vi "AlarmasHMI.vi"() -> ()   [LabVIEW 2018]
uses:
  <vilib>/RAFA Solutions/Harmony UI Controls Kit/String & Path/String Indicator.ctl
  <vilib>/RAFA Solutions/Harmony UI Controls Kit/Boolean/OK Button.ctl
  <vilib>/RAFA Solutions/Harmony UI Controls Kit/List, Table & Tree/Multicolumn Listbox.ctl
  <vilib>/RAFA Solutions/Harmony UI Controls Kit/Boolean/Blank Button - Green.ctl
  Controls/Cluster_Alarmas_IEEE45.ctl
  <vilib>/RAFA Solutions/Harmony UI Controls Kit/Boolean/Round Led.ctl
  Controls/Hora y Fecha control.ctl
  Global/globalEventos.vi
  Global/Alarmas_indicadores-LED.vi
  <vilib>/addons/database/Connection.llb/DB Tools Open Connec (Path).vi
  Global/AlarmasGlobal.vi
  <vilib>/RAFA Solutions/Harmony UI Controls Kit/Flat UI Design.lvlib
  <vilib>/addons/database/NI_Database_API.lvlib
panel:
  out "fecha y hora":T1
  out "G6_TRANS":T2 caption="Transiente"
  out "G6_SWELL":T2 caption="Swell"
  out "G6_SAG":T2 caption="Sag"
  out "G5_TRANS":T2 caption="Transiente"
  out "G5_SWELL":T2 caption="Swell"
  out "G5_SAG":T2 caption="Sag"
  out "G4_TRANS":T2 caption="Transiente"
  out "G4_SWELL":T2 caption="Swell"
  out "G4_SAG":T2 caption="Sag"
  out "G3_TRANS":T2 caption="Transiente"
  out "G3_SWELL":T2 caption="Swell"
  out "G3_SAG":T2 caption="Sag"
  out "G2_TRANS":T2 caption="Transiente"
  out "G2_SWELL":T2 caption="Swell"
  out "G2_SAG":T2 caption="Sag"
  out "G1_TRANS":T2 caption="Transiente"
  out "G1_SWELL":T2 caption="Swell"
  out "G1_SAG":T2 caption="Sag"
  out "Generador 6":T3={"V1_V2 (V) "={0.0, 17.0, 16.662651515468255}, "Mod_V1_V2"=0.0, "alarma 1"=FALSE, "Mod_V2_V3"=0.0, "alarma 2"=FALSE, "Mod_V3_V1"=0.0, "alarma 3"=FALSE, "Mod_Frec"=0.0, "alarma 4"=FALSE, "V2_V3 (V)"={0.0, 17.0, 16.662651515468255}, "V3_V1 (V)"={0.0, 17.0, 16.662651515468255}, "Frecuencia (Hz)"={0.0, 17.0, 16.662651515468255}, "AVG VL_VL (V)"={0.0, 17.0, 16.662651515468255}, "alarm 5"=FALSE, "alarm 6"=FALSE, "alarm 7"=FALSE, "alarm 8"=FALSE, "alarm 9"=FALSE} {"AVG VL_VL (V)" scale=427.0..473.0; "Frecuencia (Hz)" scale=58.0..62.0; "V3_V1 (V)" scale=418.0..482.0; "V2_V3 (V)" scale=418.0..482.0; "Mod_Frec" format="%#.1f"; "Mod_V3_V1" format="%#.1f"; "Mod_V2_V3" format="%#.1f"; "Mod_V1_V2" format="%#.1f"; "V1_V2 (V)" scale=418.0..482.0}
  out "Generador 5":T3={"V1_V2 (V) "={0.0, 17.0, 16.662651515468255}, "Mod_V1_V2"=0.0, "alarma 1"=FALSE, "Mod_V2_V3"=0.0, "alarma 2"=FALSE, "Mod_V3_V1"=0.0, "alarma 3"=FALSE, "Mod_Frec"=0.0, "alarma 4"=FALSE, "V2_V3 (V)"={0.0, 17.0, 16.662651515468255}, "V3_V1 (V)"={0.0, 17.0, 16.662651515468255}, "Frecuencia (Hz)"={0.0, 17.0, 16.662651515468255}, "AVG VL_VL (V)"={0.0, 17.0, 16.662651515468255}, "alarm 5"=FALSE, "alarm 6"=FALSE, "alarm 7"=FALSE, "alarm 8"=FALSE, "alarm 9"=FALSE} {"AVG VL_VL (V)" scale=427.0..473.0; "Frecuencia (Hz)" scale=58.0..62.0; "V3_V1 (V)" scale=418.0..482.0; "V2_V3 (V)" scale=418.0..482.0; "Mod_Frec" format="%#.1f"; "Mod_V3_V1" format="%#.1f"; "Mod_V2_V3" format="%#.1f"; "Mod_V1_V2" format="%#.1f"; "V1_V2 (V)" scale=418.0..482.0}
  out "Generador 4":T3={"V1_V2 (V) "={0.0, 17.0, 16.662651515468255}, "Mod_V1_V2"=0.0, "alarma 1"=FALSE, "Mod_V2_V3"=0.0, "alarma 2"=FALSE, "Mod_V3_V1"=0.0, "alarma 3"=FALSE, "Mod_Frec"=0.0, "alarma 4"=FALSE, "V2_V3 (V)"={0.0, 17.0, 16.662651515468255}, "V3_V1 (V)"={0.0, 17.0, 16.662651515468255}, "Frecuencia (Hz)"={0.0, 17.0, 16.662651515468255}, "AVG VL_VL (V)"={0.0, 17.0, 16.662651515468255}, "alarm 5"=FALSE, "alarm 6"=FALSE, "alarm 7"=FALSE, "alarm 8"=FALSE, "alarm 9"=FALSE} {"AVG VL_VL (V)" scale=427.0..473.0; "Frecuencia (Hz)" scale=58.0..62.0; "V3_V1 (V)" scale=418.0..482.0; "V2_V3 (V)" scale=418.0..482.0; "Mod_Frec" format="%#.1f"; "Mod_V3_V1" format="%#.1f"; "Mod_V2_V3" format="%#.1f"; "Mod_V1_V2" format="%#.1f"; "V1_V2 (V)" scale=418.0..482.0}
  out "Generador 3":T3={"V1_V2 (V) "={0.0, 17.0, 16.662651515468255}, "Mod_V1_V2"=0.0, "alarma 1"=FALSE, "Mod_V2_V3"=0.0, "alarma 2"=FALSE, "Mod_V3_V1"=0.0, "alarma 3"=FALSE, "Mod_Frec"=0.0, "alarma 4"=FALSE, "V2_V3 (V)"={0.0, 17.0, 16.662651515468255}, "V3_V1 (V)"={0.0, 17.0, 16.662651515468255}, "Frecuencia (Hz)"={0.0, 17.0, 16.662651515468255}, "AVG VL_VL (V)"={0.0, 17.0, 16.662651515468255}, "alarm 5"=FALSE, "alarm 6"=FALSE, "alarm 7"=FALSE, "alarm 8"=FALSE, "alarm 9"=FALSE} {"AVG VL_VL (V)" scale=427.0..473.0; "Frecuencia (Hz)" scale=58.0..62.0; "V3_V1 (V)" scale=418.0..482.0; "V2_V3 (V)" scale=418.0..482.0; "Mod_Frec" format="%#.1f"; "Mod_V3_V1" format="%#.1f"; "Mod_V2_V3" format="%#.1f"; "Mod_V1_V2" format="%#.1f"; "V1_V2 (V)" scale=418.0..482.0}
  out "Generador 2":T3={"V1_V2 (V) "={0.0, 17.0, 16.662651515468255}, "Mod_V1_V2"=0.0, "alarma 1"=FALSE, "Mod_V2_V3"=0.0, "alarma 2"=FALSE, "Mod_V3_V1"=0.0, "alarma 3"=FALSE, "Mod_Frec"=0.0, "alarma 4"=FALSE, "V2_V3 (V)"={0.0, 17.0, 16.662651515468255}, "V3_V1 (V)"={0.0, 17.0, 16.662651515468255}, "Frecuencia (Hz)"={0.0, 17.0, 16.662651515468255}, "AVG VL_VL (V)"={0.0, 17.0, 16.662651515468255}, "alarm 5"=FALSE, "alarm 6"=FALSE, "alarm 7"=FALSE, "alarm 8"=FALSE, "alarm 9"=FALSE} {"AVG VL_VL (V)" scale=427.0..473.0; "Frecuencia (Hz)" scale=58.0..62.0; "V3_V1 (V)" scale=418.0..482.0; "V2_V3 (V)" scale=418.0..482.0; "Mod_Frec" format="%#.1f"; "Mod_V3_V1" format="%#.1f"; "Mod_V2_V3" format="%#.1f"; "Mod_V1_V2" format="%#.1f"; "V1_V2 (V)" scale=418.0..482.0}
  out "Generador 1":T3={"V1_V2 (V) "={0.0, 17.0, 16.662651515468255}, "Mod_V1_V2"=0.0, "alarma 1"=FALSE, "Mod_V2_V3"=0.0, "alarma 2"=FALSE, "Mod_V3_V1"=0.0, "alarma 3"=FALSE, "Mod_Frec"=0.0, "alarma 4"=FALSE, "V2_V3 (V)"={0.0, 17.0, 16.662651515468255}, "V3_V1 (V)"={0.0, 17.0, 16.662651515468255}, "Frecuencia (Hz)"={0.0, 17.0, 16.662651515468255}, "AVG VL_VL (V)"={0.0, 17.0, 16.662651515468255}, "alarm 5"=FALSE, "alarm 6"=FALSE, "alarm 7"=FALSE, "alarm 8"=FALSE, "alarm 9"=FALSE} {"AVG VL_VL (V)" scale=427.0..473.0; "Frecuencia (Hz)" scale=58.0..62.0; "V3_V1 (V)" scale=418.0..482.0; "V2_V3 (V)" scale=418.0..482.0; "Mod_Frec" format="%#.1f"; "Mod_V3_V1" format="%#.1f"; "Mod_V2_V3" format="%#.1f"; "Mod_V1_V2" format="%#.1f"; "V1_V2 (V)" scale=418.0..482.0}
  in  "Tiempo Final Eventos":timestamp caption="Tiempo Final" format="%<%X\n%x>T"
  in  "Tiempo Inicio Eventos":timestamp caption="Tiempo Inicio" format="%<%X\n%x>T"
  in  "Consultar Alarma":T4
  out "Tabla de Alarmas":T5
  out "Generador":string
  in  "volver":T6
  out "Eventos":T7
  # "Sistema de Monitoreo de Calidad de Energía"
  # "Límites y valores según IEEE45"
  # "Límites y valores según IEEE45"
  # "EMCE G01"
  # "EMCE G03"
  # "EMCE G02"
  # "EMCE G04"
  # "EMCE W01"
  # "EMCE W02"
  # "ALARMAS CALIDAD DE ENERGIA\nEN50160"
  # "EMCE G03"
  # "EMCE G01"
  # "EMCE G02"
  # "EMCE W01"
  # "EMCE G04"
  # "EMCE W02"
  # "Tolerancias"
  # "Modulación"
  # "%"
  # "%"
  # "%"
  # "5 % máx."
  # "%"
  # "0,5 % máx."
  # "Tolerancias"
  # "Modulación"
  # "%"
  # "%"
  # "%"
  # "5 % máx."
  # "%"
  # "0,5 % máx."
  # "Tolerancias"
  # "Modulación"
  # "%"
  # "%"
  # "%"
  # "5 % máx."
  # "%"
  # "0,5 % máx."
  # "Tolerancias"
  # "Modulación"
  # "%"
  # "%"
  # "%"
  # "5 % máx."
  # "%"
  # "0,5 % máx."
  # "Tolerancias"
  # "Modulación"
  # "%"
  # "%"
  # "%"
  # "5 % máx."
  # "%"
  # "0,5 % máx."
  # "Tolerancias"
  # "Modulación"
  # "%"
  # "%"
  # "%"
  # "5 % máx."
  # "%"
  # "0,5 % máx."
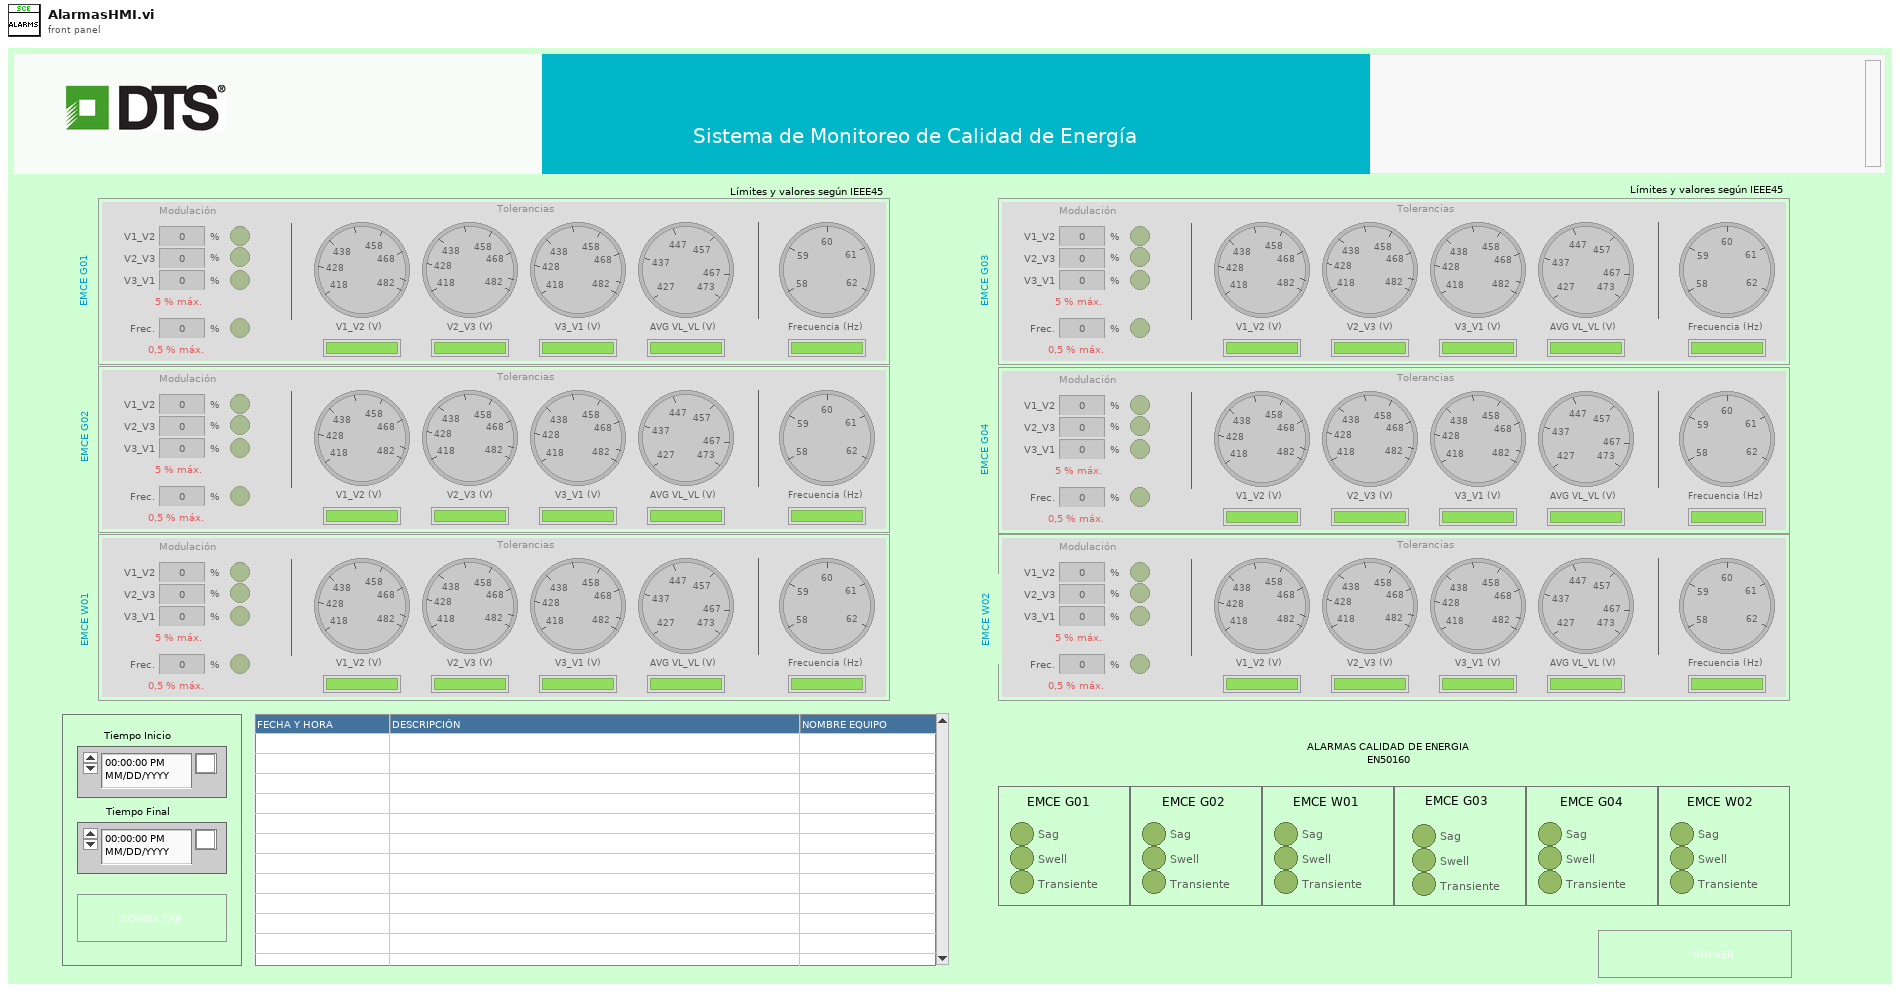
[diagram p1: front panel]
types:
  T1 = typedef "Hora y Fecha control.ctl" = cluster{"fecha":string, "dia semana":string, "fecha 2":string}
  T2 = typedef "Flat UI Design.lvlib/Round Led.ctl" = bool
  T3 = typedef "Cluster_Alarmas_IEEE45.ctl" = cluster{"V1_V2 (V) ":cluster{dbl, dbl, dbl}, "Mod_V1_V2":dbl, "alarma 1":T2, "Mod_V2_V3":dbl, "alarma 2":T2, "Mod_V3_V1":dbl, "alarma 3":T2, "Mod_Frec":dbl, "alarma 4":T2, "V2_V3 (V)":cluster{dbl, dbl, dbl}, "V3_V1 (V)":cluster{dbl, dbl, dbl}, "Frecuencia (Hz)":cluster{dbl, dbl, dbl}, "AVG VL_VL (V)":cluster{dbl, dbl, dbl}, "alarm 5":bool, "alarm 6":bool, "alarm 7":bool, "alarm 8":bool, "alarm 9":bool}
  T4 = typedef "Flat UI Design.lvlib/Blank Button - Green.ctl" = bool
  T5 = typedef "Flat UI Design.lvlib/Multicolumn Listbox.ctl" = i32
  T6 = typedef "Flat UI Design.lvlib/OK Button.ctl" = bool
  T7 = typedef "Flat UI Design.lvlib/String Indicator.ctl" = string
  T8 = typedef "NI_Database_API.lvlib/Conn ObjectReference.ctl" = refnum<k1>
  T9 = enum8{"Enabled", "Disabled", "Disabled and Grayed Out"}
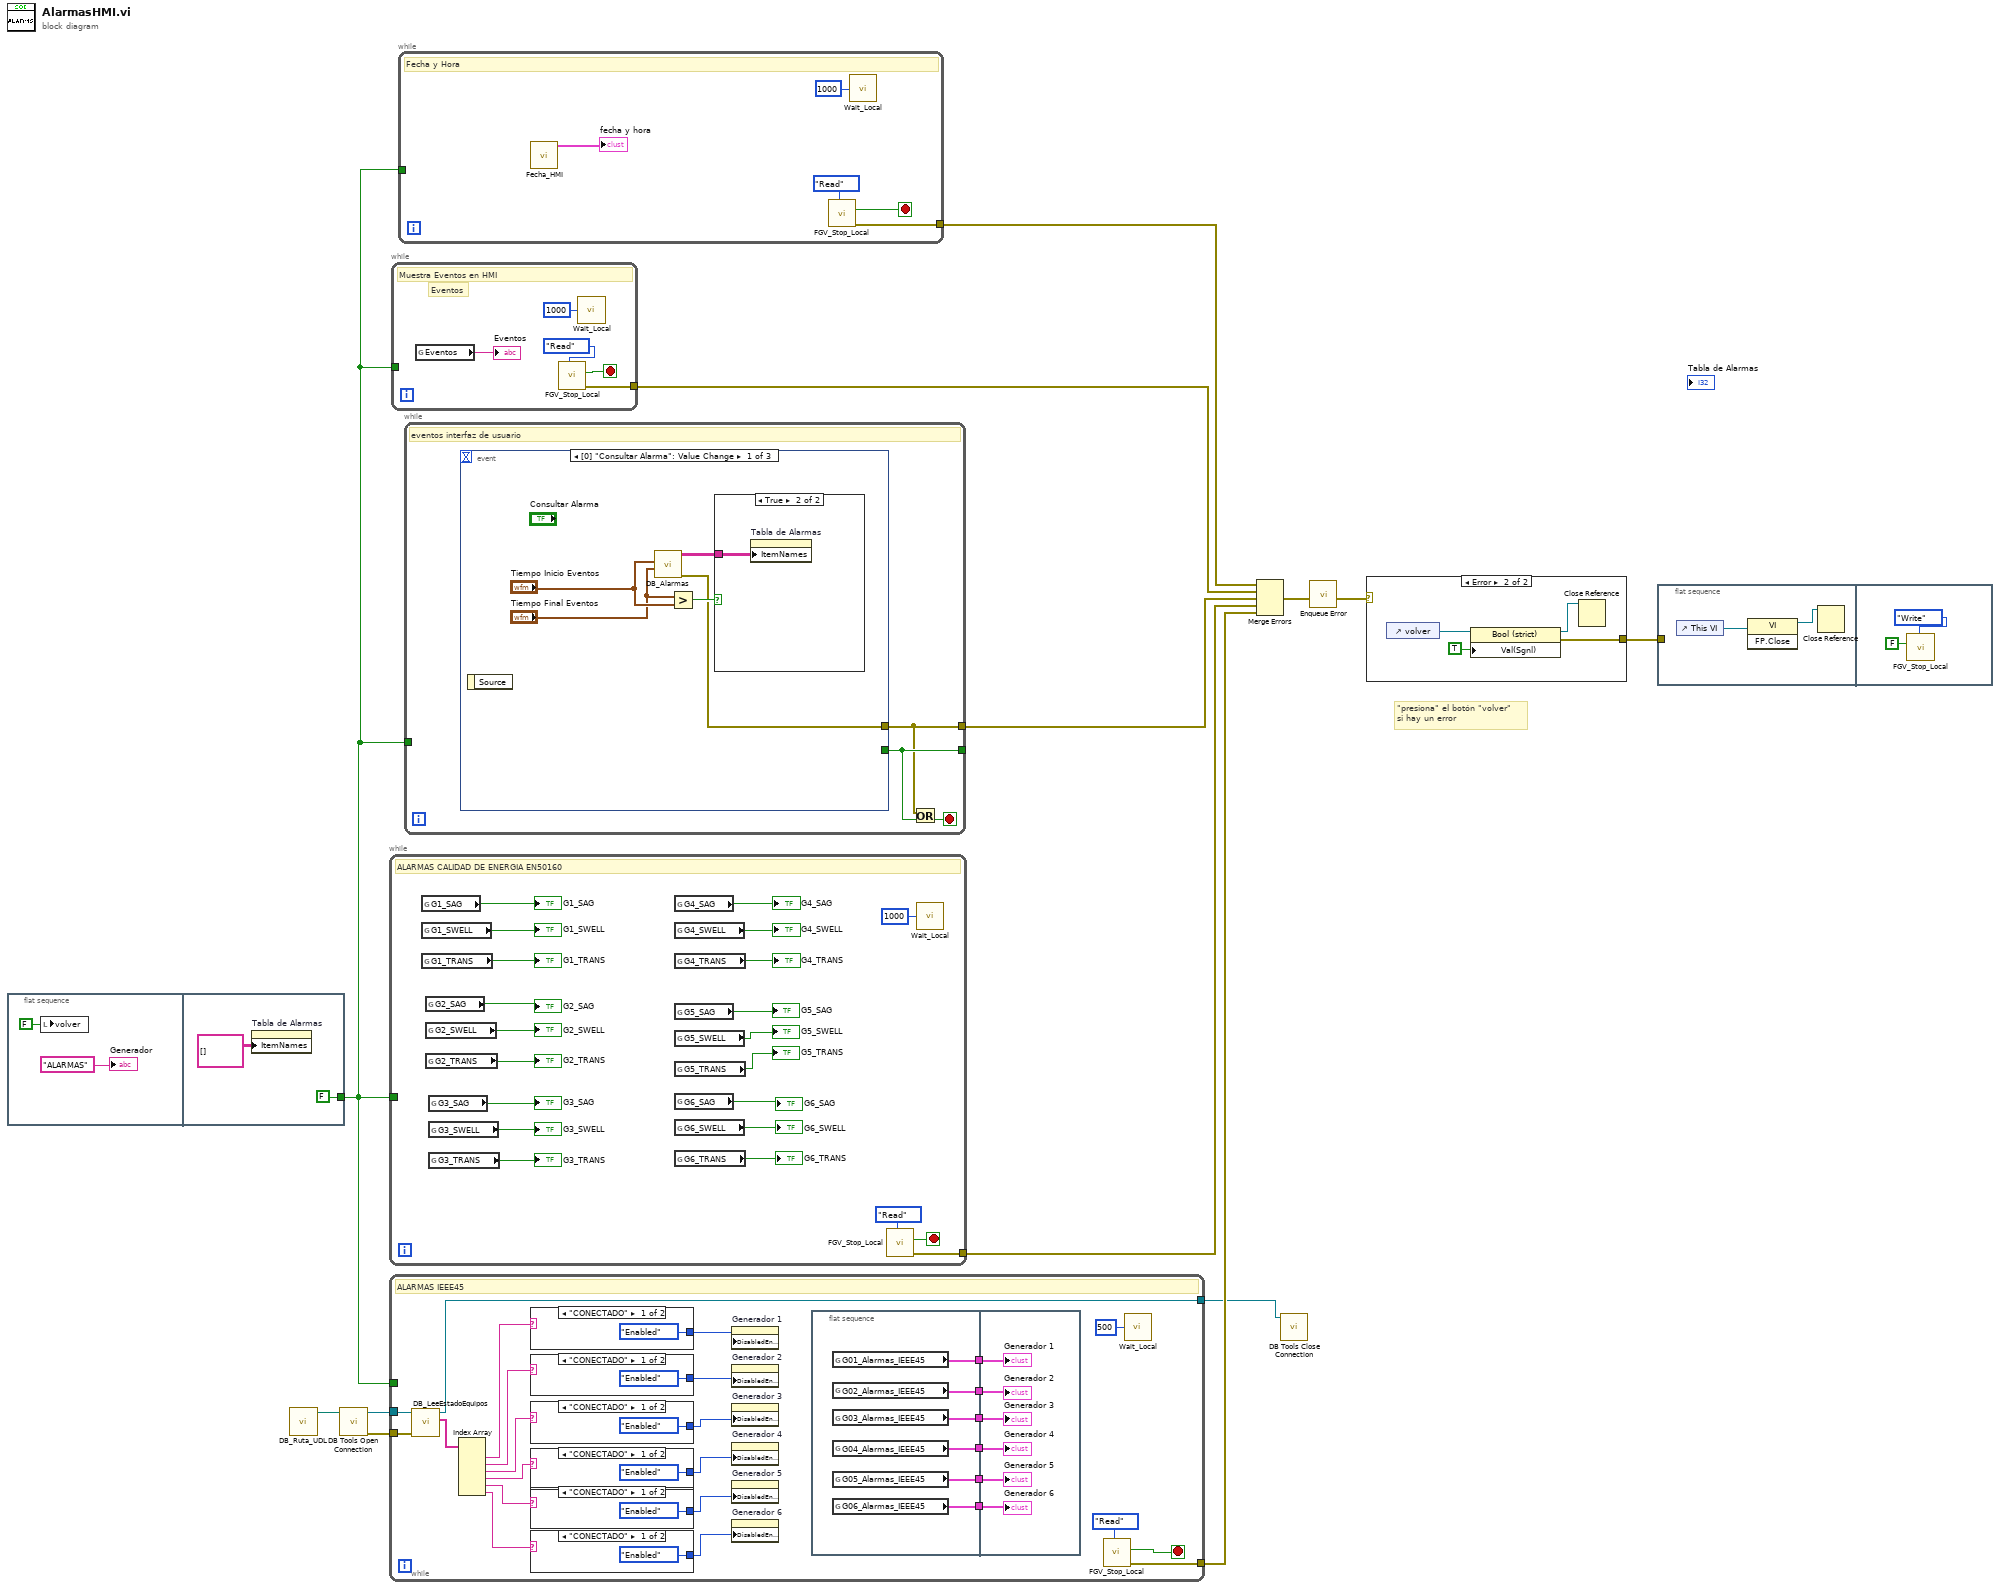
[diagram p0: block diagram]
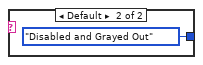
[diagram p3: hidden frame]
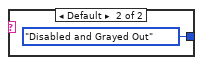
[diagram p4: hidden frame]
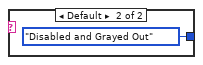
[diagram p5: hidden frame]
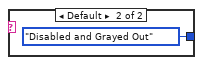
[diagram p6: hidden frame]
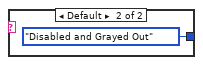
[diagram p7: hidden frame]
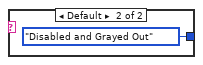
[diagram p8: hidden frame]
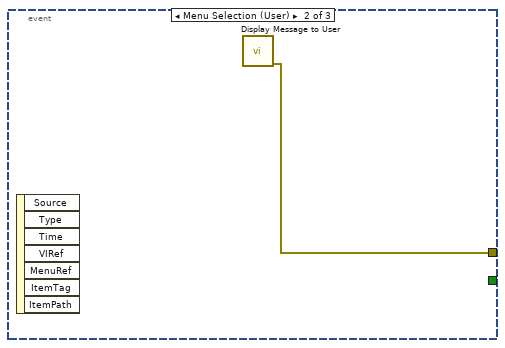
[diagram p10: hidden frame]
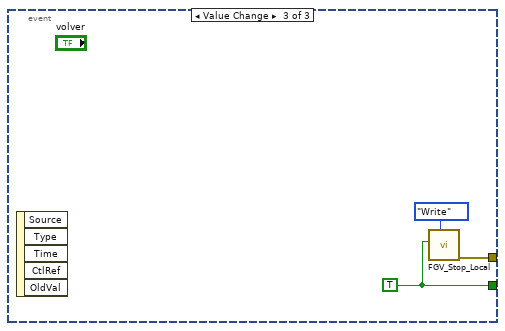
[diagram p11: hidden frame]
diagram:
  # "\"presiona\" el botón \"volver\"\nsi hay un error"
  n1 = flat-sequence {
    tunnel: [FALSE ("sag_flag")] -> w13
    frame #0 {
      n2 = local write "volver"(T6 FALSE ("volver")) -> ()
      "Generador" <- "ALARMAS" ("Generador in")
    }
    frame #1 {
      n3 = property on="Tabla de Alarmas" class="MCListbox (strict)"("ItemNames"=string[][] [] ("Item Names")) -> ()  [unwired: 2 in, 2 out]
    }
  }
  n4 = call "DB_Ruta_UDL.vi"() -> ("UDL ruta"=w4:path)  [unwired: 11 in]
  n5 = call-poly <vilib>:"DB Tools Open Connection.vi"("connection information"=w4) -> ("error out"=w3:errorcluster, "connection reference"=w2:T8)  [unwired: 7 in]
  n6 = while {
    tunnel: w13 -> [_]
    tunnel: [w36] -> w9
    stop <- w38 stop-if-true
    # "ALARMAS CALIDAD DE ENERGIA EN50160"
    n7 = global read "Alarmas_indicadores-LED.vi" "G1_SAG"() -> (→"G1_SAG":bool)
    n8 = global read "Alarmas_indicadores-LED.vi" "G1_SWELL"() -> (→"G1_SWELL":bool)
    n9 = global read "Alarmas_indicadores-LED.vi" "G1_TRANS"() -> (→"G1_TRANS":bool)
    n10 = global read "Alarmas_indicadores-LED.vi" "G2_SAG"() -> (→"G2_SAG":bool)
    n11 = global read "Alarmas_indicadores-LED.vi" "G2_SWELL"() -> (→"G2_SWELL":bool)
    n12 = global read "Alarmas_indicadores-LED.vi" "G2_TRANS"() -> (→"G2_TRANS":bool)
    n13 = global read "Alarmas_indicadores-LED.vi" "G3_SAG"() -> (→"G3_SAG":bool)
    n14 = global read "Alarmas_indicadores-LED.vi" "G3_SWELL"() -> (→"G3_SWELL":bool)
    n15 = global read "Alarmas_indicadores-LED.vi" "G3_TRANS"() -> (→"G3_TRANS":bool)
    n16 = global read "Alarmas_indicadores-LED.vi" "G4_SAG"() -> (→"G4_SAG":bool)
    n17 = global read "Alarmas_indicadores-LED.vi" "G4_SWELL"() -> (→"G4_SWELL":bool)
    n18 = global read "Alarmas_indicadores-LED.vi" "G4_TRANS"() -> (→"G4_TRANS":bool)
    n19 = global read "Alarmas_indicadores-LED.vi" "G5_SAG"() -> (→"G5_SAG":bool)
    n20 = global read "Alarmas_indicadores-LED.vi" "G5_SWELL"() -> (→"G5_SWELL":bool)
    n21 = global read "Alarmas_indicadores-LED.vi" "G5_TRANS"() -> (→"G5_TRANS":bool)
    n22 = global read "Alarmas_indicadores-LED.vi" "G6_SAG"() -> (→"G6_SAG":bool)
    n23 = global read "Alarmas_indicadores-LED.vi" "G6_SWELL"() -> (→"G6_SWELL":bool)
    n24 = global read "Alarmas_indicadores-LED.vi" "G6_TRANS"() -> (→"G6_TRANS":bool)
    n25 = call "FGV_Stop_Local.vi"("Action"=enum16{"Read", "Write"}."Read") -> ("Error Out"=w36:errorcluster, "Var Out"=w38:bool)  [unwired: 9 in]
    n26 = call "Wait_Local.vi"("Wait time (msec)"=u32 1000) -> ()  [unwired: 5 in]
  }
  n27 = while {
    tunnel: w13 -> [_]
    tunnel: [w63] -> w8
    tunnel: w3 -> [w55]
    tunnel: w2 -> [w54]
    tunnel: [w40] -> w1
    stop <- w65 stop-if-true
    # "ALARMAS IEEE45"
    n28 = call "DB_LeeEstadoEquipos.vi"("error in (no error)"=w55, "db in"=w54) -> ("ESTADO_EQUIPOS"=w41:string[], "db out"=w40:T8)  [unwired: 7 in, 1 out]
    n29 = Index Array(array=w41) -> (element #1=w52:string, element #2=w51:string, element #3=w50:string, element #4=w49:string, element #5=w48:string, element #6=w47:string)  [unwired: 6 in]
    n30 = case shown="\"CONECTADO\"" w52 {
      tunnel: [T9."Enabled" ("Disabled") T9."Disabled and Grayed Out" ("Disabled")] -> w53
      frame "CONECTADO" {
      }
      frame Default {
      }
    }
    n31 = case shown="\"CONECTADO\"" w51 {
      tunnel: [T9."Enabled" ("Disabled") T9."Disabled and Grayed Out" ("Disabled")] -> w46
      frame "CONECTADO" {
      }
      frame Default {
      }
    }
    n32 = case shown="\"CONECTADO\"" w50 {
      tunnel: [T9."Enabled" ("Disabled") T9."Disabled and Grayed Out" ("Disabled")] -> w45
      frame "CONECTADO" {
      }
      frame Default {
      }
    }
    n33 = case shown="\"CONECTADO\"" w49 {
      tunnel: [T9."Enabled" ("Disabled") T9."Disabled and Grayed Out" ("Disabled")] -> w44
      frame "CONECTADO" {
      }
      frame Default {
      }
    }
    n34 = case shown="\"CONECTADO\"" w48 {
      tunnel: [T9."Enabled" ("Disabled") T9."Disabled and Grayed Out" ("Disabled")] -> w43
      frame "CONECTADO" {
      }
      frame Default {
      }
    }
    n35 = case shown="\"CONECTADO\"" w47 {
      tunnel: [T9."Enabled" ("Disabled") T9."Disabled and Grayed Out" ("Disabled")] -> w42
      frame "CONECTADO" {
      }
      frame Default {
      }
    }
    n36 = property on="Generador 1" class="Clust (strict)"("DisabledEnum"=w53) -> ()  [unwired: 2 in, 2 out]
    n37 = property on="Generador 2" class="Clust (strict)"("DisabledEnum"=w46) -> ()  [unwired: 2 in, 2 out]
    n38 = property on="Generador 3" class="Clust (strict)"("DisabledEnum"=w45) -> ()  [unwired: 2 in, 2 out]
    n39 = property on="Generador 4" class="Clust (strict)"("DisabledEnum"=w44) -> ()  [unwired: 2 in, 2 out]
    n40 = property on="Generador 5" class="Clust (strict)"("DisabledEnum"=w43) -> ()  [unwired: 2 in, 2 out]
    n41 = property on="Generador 6" class="Clust (strict)"("DisabledEnum"=w42) -> ()  [unwired: 2 in, 2 out]
    n42 = flat-sequence {
      tunnel: [w83] -> w62
      tunnel: [w82] -> w61
      tunnel: [w81] -> w60
      tunnel: [w80] -> w59
      tunnel: [w79] -> w58
      tunnel: [w78] -> w57
      tunnel: w62 -> [w88]
      tunnel: w61 -> [w89]
      tunnel: w60 -> [w87]
      tunnel: w59 -> [w86]
      tunnel: w58 -> [w85]
      tunnel: w57 -> [w84]
      frame #0 {
        n43 = global read "AlarmasGlobal.vi" "G01_Alarmas_IEEE45"() -> (w82:T3)
        n44 = global read "AlarmasGlobal.vi" "G02_Alarmas_IEEE45"() -> (w83:T3)
        n45 = global read "AlarmasGlobal.vi" "G03_Alarmas_IEEE45"() -> (w81:T3)
        n46 = global read "AlarmasGlobal.vi" "G04_Alarmas_IEEE45"() -> (w80:T3)
        n47 = global read "AlarmasGlobal.vi" "G05_Alarmas_IEEE45"() -> (w79:T3)
        n48 = global read "AlarmasGlobal.vi" "G06_Alarmas_IEEE45"() -> (w78:T3)
      }
      frame #1 {
        "Generador 1" <- w89
        "Generador 2" <- w88
        "Generador 3" <- w87
        "Generador 4" <- w86
        "Generador 5" <- w85
        "Generador 6" <- w84
      }
    }
    n49 = call "FGV_Stop_Local.vi"("Action"=enum16{"Read", "Write"}."Read") -> ("Error Out"=w63:errorcluster, "Var Out"=w65:bool)  [unwired: 9 in]
    n50 = call "Wait_Local.vi"("Wait time (msec)"=u32 500 ("millisecond multiple")) -> ()  [unwired: 5 in]
  }
  n51 = while {
    tunnel: w13 -> [_]
    tunnel: [w91] -> w11
    stop <- w92 stop-if-true
    # "Eventos"
    # "Muestra Eventos en HMI"
    n52 = global read "globalEventos.vi" "Eventos"() -> (→"Eventos":string)
    n53 = call "FGV_Stop_Local.vi"("Action"=enum16{"Read", "Write"}."Read") -> ("Error Out"=w91:errorcluster, "Var Out"=w92:bool)  [unwired: 9 in]
    n54 = call "Wait_Local.vi"("Wait time (msec)"=u32 1000 ("milliseconds to wait")) -> ()  [unwired: 5 in]
  }
  n55 = while {
    tunnel: w13 -> [_]
    tunnel: [w96] -> w12
    stop <- w97 stop-if-true
    # "Fecha y Hora"
    n56 = call "Fecha_HMI.vi"() -> ("fecha y hora"=→"fecha y hora":T1)  [unwired: 11 in]
    n57 = call "FGV_Stop_Local.vi"("Action"=enum16{"Read", "Write"}."Read") -> ("Error Out"=w96:errorcluster, "Var Out"=w97:bool)  [unwired: 9 in]
    n58 = call "Wait_Local.vi"("Wait time (msec)"=u32 1000 ("milliseconds to wait")) -> ()  [unwired: 5 in]
  }
  n59 = while {
    tunnel: [w102] -> _
    tunnel: w13 -> [_]
    tunnel: [w100] -> w10
    stop <- w101 stop-if-true
    # "eventos interfaz de usuario"
    n60 = event shown="[0] \"Consultar Alarma\": Value Change" {
      selector: _ -> [_ _ _]
      dyn-events: _ -> [_ _ _]
      timeout: _ -> [_ _ _]
      tunnel: [_ _ w111] -> w102
      tunnel: [w103 w109 w110] -> w100
      event Value Change {
        n61 = event-data() -> ()  [unwired: 1 in, 1 out]
        n62 = call "DB_Alarmas.vi"("Final"="Tiempo Final Eventos", "Inicio"="Tiempo Inicio Eventos") -> ("error out"=w103:errorcluster, "Data"=w107:string[][])  [unwired: 8 in]
        n63 = Greater?(x="Tiempo Final Eventos", y="Tiempo Inicio Eventos") -> (0:w104:bool)
        n64 = case shown="True" w104 {
          tunnel: w107 -> [_ w108]
          frame False {
            # "#ToDo Alarma\nPoner dialogo"
          }
          frame True {
            n65 = property on="Tabla de Alarmas" class="MCListbox (strict)"("ItemNames"=w108) -> ()  [unwired: 2 in, 2 out]
          }
        }
      }
      event Menu Selection (User) {
        n66 = event-data() -> ()  [unwired: 1 in, 7 out]
        n67 = call "Display Message to User"() -> ("error out"=w109:errorcluster)  [unwired: 10 in, 1 out]
      }
      event Value Change {
        w111 = TRUE
        n68 = event-data() -> ()  [unwired: 1 in, 5 out]
        n69 = call "FGV_Stop_Local.vi"("Action"=enum16{"Read", "Write"}."Write", "Var In"=w111) -> ("Error Out"=w110:errorcluster)  [unwired: 8 in, 1 out]
      }
    }
    n70 = Or(x=w100, y=w102) -> (x .or. y?=w101:bool)
  }
  n71 = Merge Errors(w12, w11, w10, w9, w8) -> (w7:errorcluster)
  n72 = call <vilib>:"DB Tools Close Connection.vi"("connection reference"=w1) -> ()  [unwired: 6 in, 1 out]
  n73 = call "Enqueue Error.vi"("error in"=w7) -> ("error out"=w5:errorcluster)  [unwired: 9 in, 1 out]
  n74 = case shown="Error" w5 {
    selector: w5 -> [w113 _]
    tunnel: [w113 w115] -> w6
    frame No Error {
    }
    frame Error {
      n75 = control-ref of="volver"() -> (w117:refnum<vi>)
      n76 = property class="Bool (strict)"(reference=w117, "Val(Sgnl)"=TRUE) -> (reference out=w114:refnum<vi>, error out=w115:errorcluster)  [unwired: 1 in]
      n77 = Close Reference(reference=w114) -> ()  [unwired: 1 in, 1 out]
    }
  }
  n78 = flat-sequence {
    tunnel: w6 -> [_]
    frame #0 {
      n79 = control-ref of="This VI"() -> (w119:refnum<vi>)
      n80 = invoke class="VI" method="FP.Close"(reference=w119) -> (reference out=w118:refnum<vi>)  [unwired: 2 in, 2 out]
      n81 = Close Reference(reference=w118) -> ()  [unwired: 1 in, 1 out]
    }
    frame #1 {
      n82 = call "FGV_Stop_Local.vi"("Action"=enum16{"Read", "Write"}."Write", "Var In"=FALSE) -> ()  [unwired: 8 in, 2 out]
    }
  }
